vi "Initialize Protection Frames Outgoing.vi"(8 "error in (no error)":errorcluster, 10 "Frames":T1[](array[typedef]) {"Protection Configurations"."CRC Channels"."Data Type" items=["Signed", "Unsigned", "IEEE Float"]}, 11 "PCL (usec)":u32) -> (0 "error out":errorcluster, 2 "RT Frames":T8[](array[typedef]) {"Protection Configurations"."CRC Channels"."Data Type" items=["Signed", "Unsigned", "IEEE Float"]})   [LabVIEW 2023, in "Protection and Counter Support Engine.lvlib"]
uses:
  Protection and Counter Support Engine.lvlib
  Types/RT Frame Settings.ctl
  Shared/Types/Exported Frame Type.ctl
  Types/RT Protection Configuration.ctl
  Shared/Types/Protection Type.ctl
  Shared/Types/XNET Signal Configuration.ctl
  Shared/Types/Exported Counter Settings.ctl
  Shared/Types/Exported Event Trigger Type.ctl
  Shared/Types/Exported Frame Settings.ctl
  Shared/Types/Exported Protection Settings.ctl
  <vilib>/xnet/xnet.llb/XNET Create Session (Conversion).vi
  Shared/Protection and Counter Support Shared.lvlib
  LP_CRC/LP_CRC.lvlib
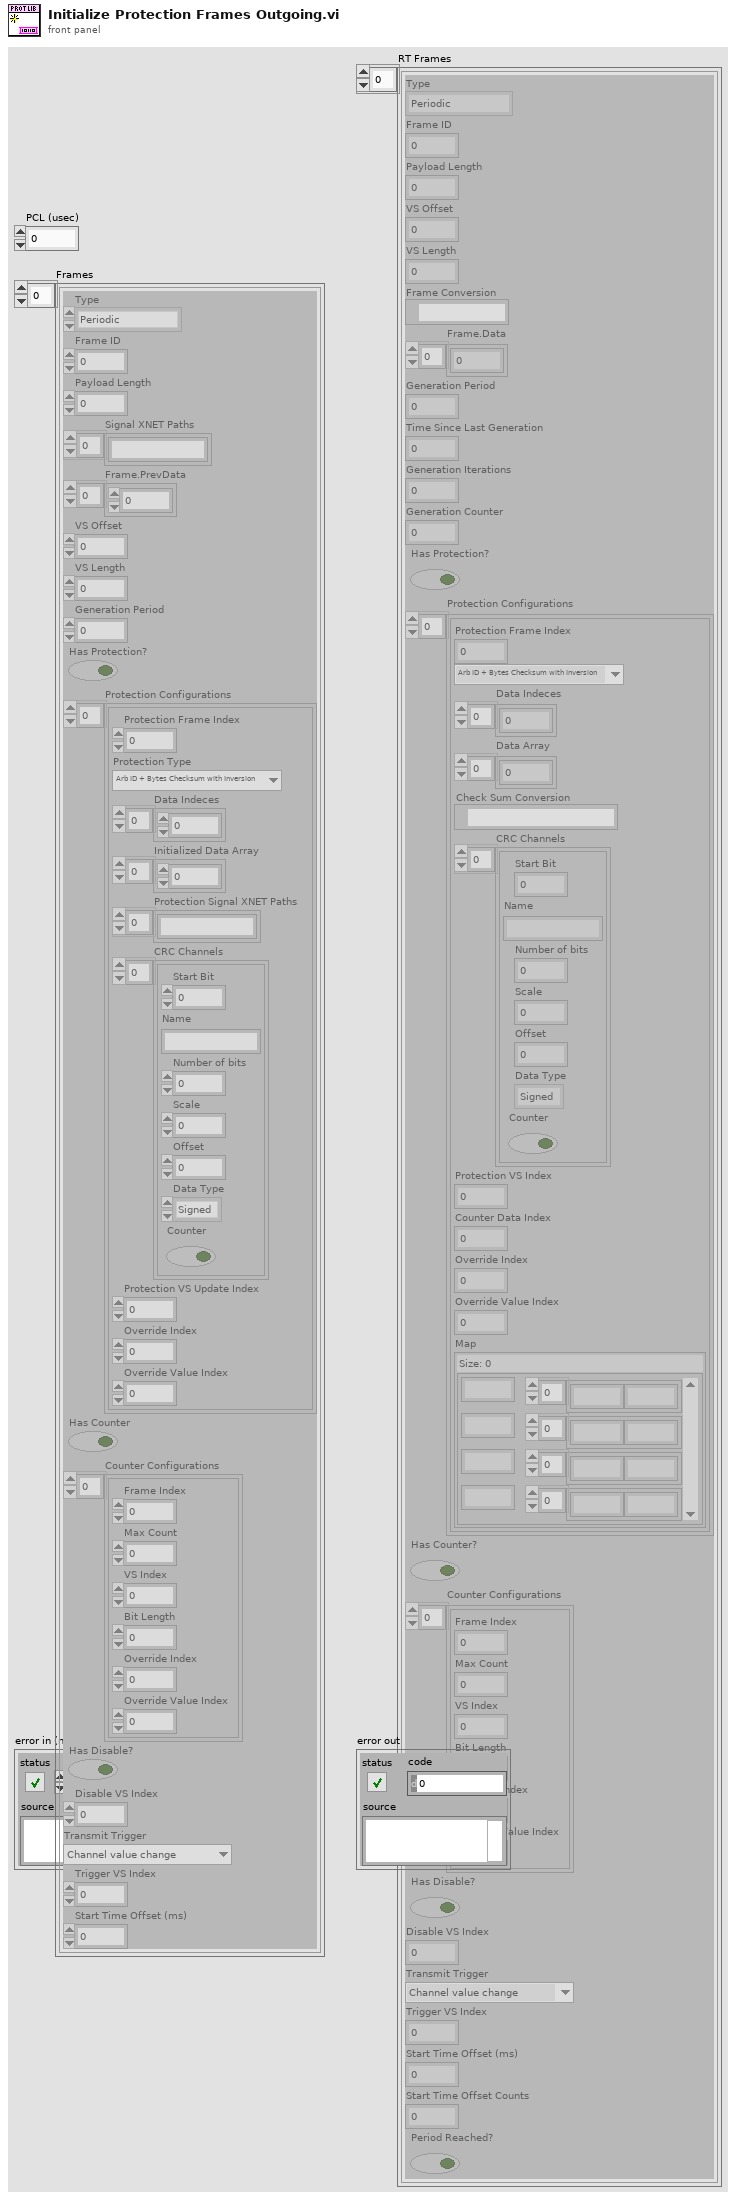
[diagram p1: front panel]
types:
  T1 = typedef "Protection and Counter Support Shared.lvlib/Exported Frame Settings.ctl" = cluster{"Type":T2, "Frame ID":u32, "Payload Length":u32, "Signal XNET Paths":string[], "Frame.PrevData":dbl[], "VS Offset":i32, "VS Length":i32, "Generation Period":u32, "Has Protection?":bool, "Protection Configurations":T3[], "Has Counter":bool, "Counter Configurations":T6[], "Has Disable?":bool, "Disable VS Index":i32, "Transmit Trigger":T7, "Trigger VS Index":i32, "Start Time Offset (ms)":u32}
  T2 = typedef "Protection and Counter Support Shared.lvlib/Exported Frame Type.ctl" = enum16{"Periodic", "Event", "Periodic/Event"}
  T3 = typedef "Protection and Counter Support Shared.lvlib/Exported Protection Settings.ctl" = cluster{"Protection Frame Index":i32, "Protection Type":T4, "Data Indeces":i32[], "Initialized Data Array":dbl[], "Protection Signal XNET Paths":string[], "CRC Channels":T5[], "Protection VS Update Index":i32, "Override Index":i32, "Override Value Index":i32}
  T4 = typedef "Protection and Counter Support Shared.lvlib/Protection Type.ctl" = enum16{"Arb ID + Bytes Checksum with Inversion", "Arb ID + Bytes CRC with Inversion", "Reversed Raw Signal Checksum with Inversion", "Concatenated Two's Compliment", "LP_CRC8", "LP_Checksum", "LP_CRC8_MRS"}
  T5 = typedef "Protection and Counter Support Shared.lvlib/XNET Signal Configuration.ctl" = cluster{"Start Bit":i32, "Name":string, "Number of bits":i32, "Scale":dbl, "Offset":dbl, "Data Type":u32, "Counter":bool}
  T6 = typedef "Protection and Counter Support Shared.lvlib/Exported Counter Settings.ctl" = cluster{"Frame Index":i32, "Max Count":dbl, "VS Index":i32, "Bit Length":i64, "Override Index":i32, "Override Value Index":i32}
  T7 = typedef "Protection and Counter Support Shared.lvlib/Exported Event Trigger Type.ctl" = enum16{"Channel value change", "Trigger channel (not zero)", "Channel value change or trigger channel (not zero)", "Trigger channel (any value change)", "Channel value change or trigger channel (any value change)"}
  T8 = typedef "Protection and Counter Support Engine.lvlib/RT Frame Settings.ctl" = cluster{"Type":T2, "Frame ID":u32, "Payload Length":u32, "VS Offset":i32, "VS Length":i32, "Frame Conversion":refnum<k21>, "Frame.Data":dbl[], "Generation Period":u32, "Time Since Last Generation":u32, "Generation Iterations":u32, "Generation Counter":u32, "Has Protection?":bool, "Protection Configurations":T9[], "Has Counter?":bool, "Counter Configurations":T6[], "Has Disable?":bool, "Disable VS Index":i32, "Transmit Trigger":T7, "Trigger VS Index":i32, "Start Time Offset (ms)":u32, "Start Time Offset Counts":u32, "Period Reached?":bool}
  T9 = typedef "Protection and Counter Support Engine.lvlib/RT Protection Configuration.ctl" = cluster{"Protection Frame Index":i32, "Protection Type":T4, "Data Indeces":i32[], "Data Array":dbl[], "Check Sum Conversion":refnum<k21>, "CRC Channels":T5[], "Protection VS Index":i32, "Counter Data Index":i32, "Override Index":i32, "Override Value Index":i32, "Map":map{i32, u8[]}}
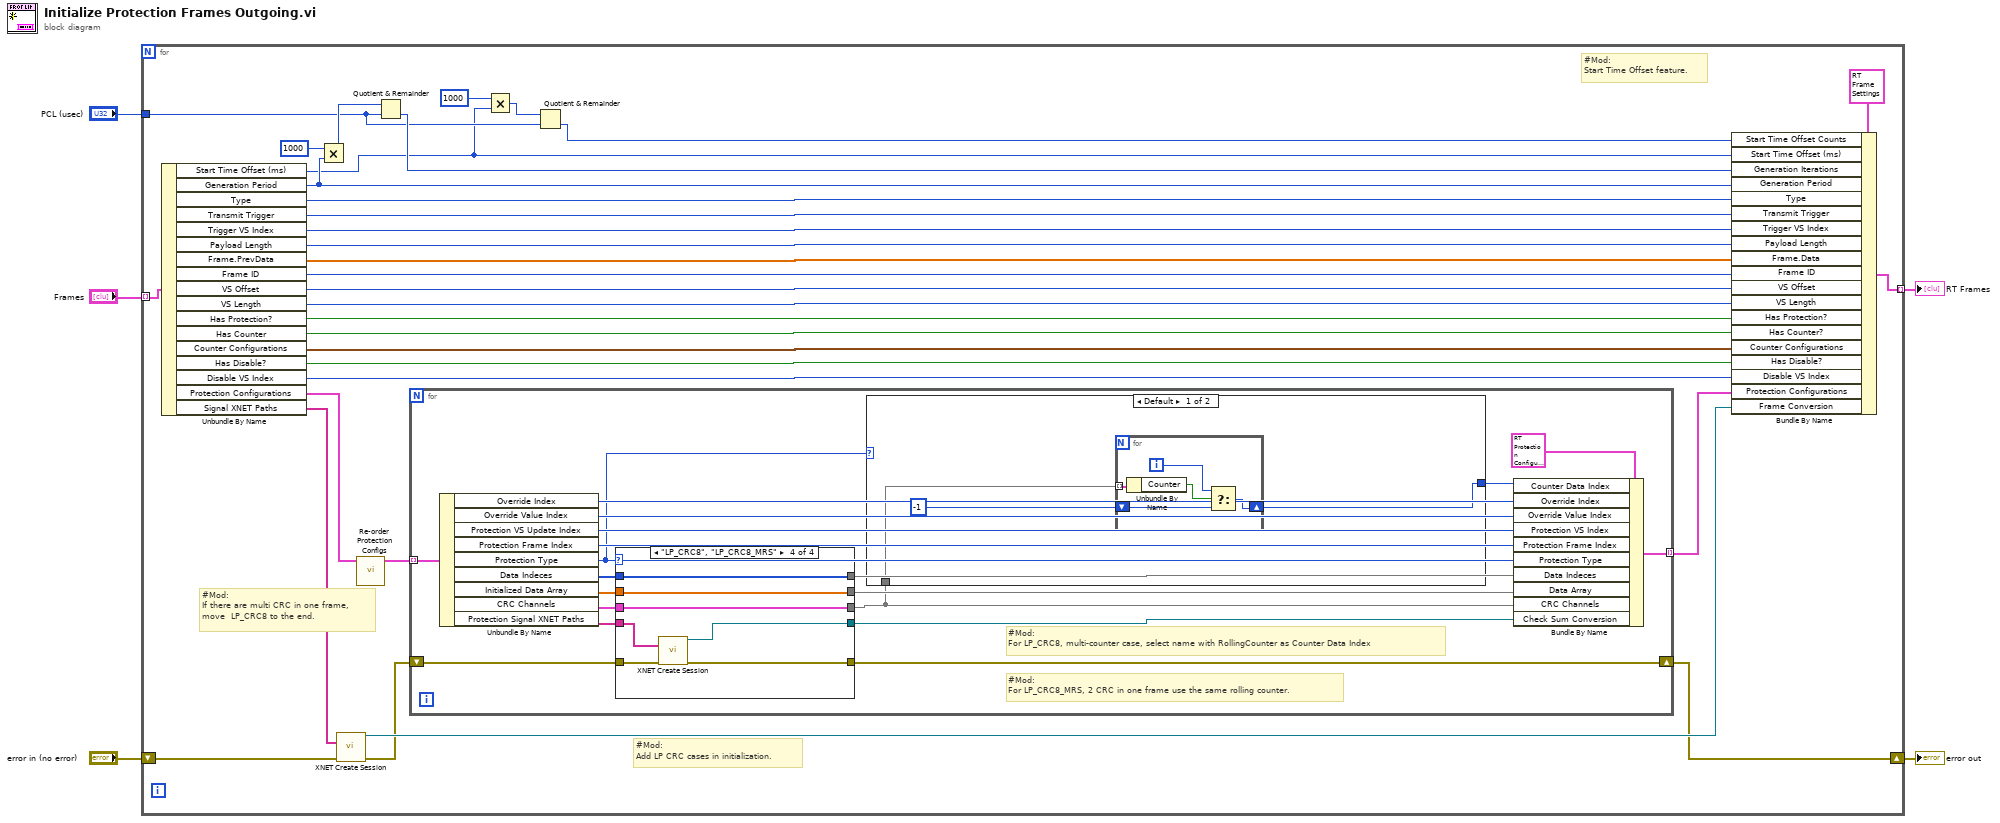
[diagram p0: block diagram]
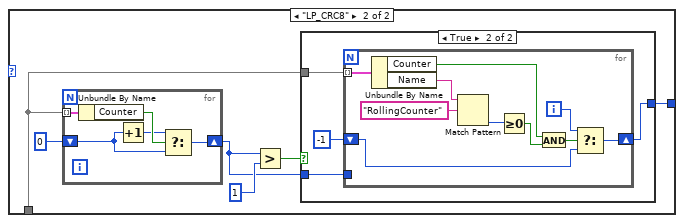
[diagram p2: hidden frame]
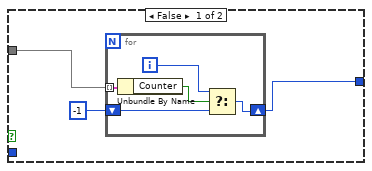
[diagram p3: hidden frame]
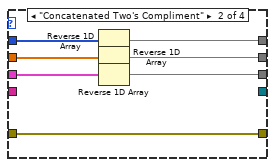
[diagram p5: hidden frame]
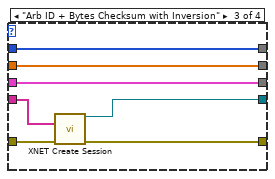
[diagram p6: hidden frame]
diagram:
  n1 = for {
    shift-right: [w24] -> w3
    shift-left: "error in (no error)" -> [w36]
    tunnel: "Frames" -> [w38] mode=indexing
    tunnel: [w23] -> w1 mode=indexing
    tunnel: "PCL (usec)" -> [w8]
    # "#Mod:\nStart Time Offset feature."
    # "#Mod:\nAdd LP CRC cases in initialization."
    # "#Mod:\nIf there are multi CRC in one frame,\nmove  LP_CRC8 to the end."
    n2 = Unbundle By Name(w38) -> ("Start Time Offset (ms)"=w6:u32, "Generation Period"=w18:u32, "Type"=w13:T2, "Transmit Trigger"=w14:T7, "Trigger VS Index"=w15:i32, "Payload Length"=w16:u32, "Frame.PrevData"=w21:dbl[], "Frame ID"=w34:u32, "VS Offset"=w33:i32, "VS Length"=w32:i32, "Has Protection?"=w31:bool, "Has Counter"=w30:bool, "Counter Configurations"=w29:T6[], "Has Disable?"=w28:bool, "Disable VS Index"=w27:i32, "Protection Configurations"=w11:T3[], "Signal XNET Paths"=w37:string[])
    n3 = Multiply(x=u32 1000, y=w18) -> (x*y=w19:u32)
    n4 = call-poly <vilib>:"XNET Create Session.vi"("signal list"=w37, "error in (no error)"=w36) -> ("session out"=w35:refnum<k21>, "error out"=w25:errorcluster)  [unwired: 12 out]
    n5 = call "Re-order Protection Configs.vi"("Protection Configurations"=w11) -> ("Protection Configurations Out"=w12:T3[])  [unwired: 10 in]
    n6 = Quotient & Remainder(x=w19, y=w8) -> (floor(x/y)=w17:u32)  [unwired: 1 out]
    n7 = for {
      tunnel: w12 -> [w57] mode=indexing
      tunnel: [w52] -> w26 mode=indexing
      shift-right: [w50] -> w24
      shift-left: w25 -> [w51]
      # "#Mod:\nFor LP_CRC8_MRS, 2 CRC in one frame use the same rolling counter."
      # "#Mod:\nFor LP_CRC8, multi-counter case, select name with RollingCounter as Counter Data Index"
      n8 = Unbundle By Name(w57) -> ("Override Index"=w43:i32, "Override Value Index"=w42:i32, "Protection VS Update Index"=w44:i32, "Protection Frame Index"=w55:i32, "Protection Type"=w41:T4, "Data Indeces"=w45:i32[], "Initialized Data Array"=w47:dbl[], "CRC Channels"=w49:T5[], "Protection Signal XNET Paths"=w54:string[])
      n9 = case shown="\"LP_CRC8\", \"LP_CRC8_MRS\"" w41 {
        tunnel: w54 -> [_ _ w116 w123]
        tunnel: [_ _ w115 w122] -> w53
        tunnel: w51 -> [w102 w109 w114 w121]
        tunnel: [w102 w109 w113 w120] -> w50
        tunnel: [w101 w105 w112 w119] -> w40
        tunnel: w49 -> [w101 w108 w112 w119]
        tunnel: [w100 w104 w111 w118] -> w48
        tunnel: w47 -> [w100 w107 w111 w118]
        tunnel: [w99 w103 w110 w117] -> w46
        tunnel: w45 -> [w99 w106 w110 w117]
        frame Default {
        }
        frame "Concatenated Two's Compliment" {
          n10 = Reverse 1D Array(array=w106) -> (reversed array=w103:i32[])
          n11 = Reverse 1D Array(array=w107) -> (reversed array=w104:dbl[])
          n12 = Reverse 1D Array(array=w108) -> (reversed array=w105:T5[])
        }
        frame "Arb ID + Bytes Checksum with Inversion" {
          n13 = call-poly <vilib>:"XNET Create Session.vi"("signal list"=w116, "error in (no error)"=w114) -> ("session out"=w115:refnum<k21>, "error out"=w113:errorcluster)  [unwired: 12 out]
        }
        frame "LP_CRC8", "LP_CRC8_MRS" {
          n14 = call-poly <vilib>:"XNET Create Session.vi"("signal list"=w123, "error in (no error)"=w121) -> ("session out"=w122:refnum<k21>, "error out"=w120:errorcluster)  [unwired: 12 out]
        }
      }
      n15 = case shown="Default" w41 {
        tunnel: w40 -> [w59 w69]
        tunnel: [w58 w70] -> w39
        frame Default {
          n16 = for {
            tunnel: w59 -> [w65] mode=indexing
            shift-right: [w61] -> w58
            shift-left: -1 -> [w63]
            i -> [w62]
            n17 = Unbundle By Name(w65) -> ("Counter"=w64:bool)
            n18 = Select(t=w62, s=w64, f=w63) -> (s? t:f=w61:i32)
          }
        }
        frame "LP_CRC8" {
          n19 = for {
            tunnel: w69 -> [w76] mode=indexing
            shift-right: [w74] -> w66
            shift-left: 0 -> [w72]
            n20 = Unbundle By Name(w76) -> ("Counter"=w75:bool)
            n21 = Increment(x=w72) -> (x+1=w73:i32)
            n22 = Select(t=w73, s=w75, f=w72) -> (s? t:f=w74:i32)
          }
          n23 = Greater?(x=w66, y=1) -> (0:w71:bool)
          n24 = case shown="True" w71 {
            tunnel: w69 -> [w78 w88]
            tunnel: [w77 w86] -> w70
            tunnel: w66 -> [_ w85]
            frame False {
              n25 = for {
                tunnel: w78 -> [w84] mode=indexing
                shift-right: [w80] -> w77
                shift-left: -1 -> [w82]
                i -> [w81]
                n26 = Unbundle By Name(w84) -> ("Counter"=w83:bool)
                n27 = Select(t=w81, s=w83, f=w82) -> (s? t:f=w80:i32)
              }
            }
            frame True {
              n28 = for {
                tunnel: w88 -> [w98] mode=indexing
                shift-right: [w93] -> w86
                shift-left: -1 -> [w90]
                tunnel: w85 -> [_]
                i -> [w91]
                n29 = Unbundle By Name(w98) -> ("Counter"=w95:bool, "Name"=w89:string)
                n30 = Match Pattern(string=w89, regular expression="RollingCounter") -> (offset past match=w96:i32)  [unwired: 1 in, 3 out]
                n31 = Greater Or Equal To 0?(x=w96) -> (x >= 0?=w94:bool)
                n32 = And(x=w95, y=w94) -> (x .and. y?=w92:bool)
                n33 = Select(t=w91, s=w92, f=w90) -> (s? t:f=w93:i32)
              }
            }
          }
        }
      }
      n34 = Bundle By Name(cluster=T9 {"Protection Frame Index"=0, "Protection Type"=enum."Arb ID + Bytes Checksum with Inversion", "Data Indeces"=[], "Data Array"=[], "Check Sum Conversion"="", "CRC Channels"=[], "Protection VS Index"=0, "Counter Data Index"=0, "Override Index"=0, "Override Value Index"=0, "Map"={}} ("Cluster"), "Counter Data Index"=w39, "Override Index"=w43, "Override Value Index"=w42, "Protection VS Index"=w44, "Protection Frame Index"=w55, "Protection Type"=w41, "Data Indeces"=w46, "Data Array"=w48, "CRC Channels"=w40, "Check Sum Conversion"=w53) -> (w52:T9)
    }
    n35 = Multiply(x=u32 1000, y=w6) -> (x*y=w9:u32)
    n36 = Quotient & Remainder(x=w9, y=w8) -> (floor(x/y)=w7:u32)  [unwired: 1 out]
    n37 = Bundle By Name(cluster=T8 {"Type"=enum."Periodic", "Frame ID"=0, "Payload Length"=0, "VS Offset"=0, "VS Length"=0, "Frame Conversion"="", "Frame.Data"=[], "Generation Period"=0, "Time Since Last Generation"=0, "Generation Iterations"=0, "Generation Counter"=0, "Has Protection?"=FALSE, "Protection Configurations"=[], "Has Counter?"=FALSE, "Counter Configurations"=[], "Has Disable?"=FALSE, "Disable VS Index"=0, "Transmit Trigger"=enum."Channel value change", "Trigger VS Index"=0, "Start Time Offset (ms)"=0, "Start Time Offset Counts"=0, "Period Reached?"=FALSE} ("Frame Settings"), "Start Time Offset Counts"=w7, "Start Time Offset (ms)"=w6, "Generation Iterations"=w17, "Generation Period"=w18, "Type"=w13, "Transmit Trigger"=w14, "Trigger VS Index"=w15, "Payload Length"=w16, "Frame.Data"=w21, "Frame ID"=w34, "VS Offset"=w33, "VS Length"=w32, "Has Protection?"=w31, "Has Counter?"=w30, "Counter Configurations"=w29, "Has Disable?"=w28, "Disable VS Index"=w27, "Protection Configurations"=w26, "Frame Conversion"=w35) -> (w23:T8)
  }
  "RT Frames" <- w1
  "error out" <- w3
